vi "AuMT8852B Password.vi"(5 "New password (0)":i32, 7 "Old password (0)":i32, 8 "error in (no error)":errorcluster, 11 "VISA session":refnum<visa-resource-name>) -> (0 "error out":errorcluster, 2 "error code":i32, 3 "VISA session out":refnum<visa-resource-name>)   [LabVIEW 2017]
doc: "Anritsu MT8852B Bluetooth Tester\n\nSets the password used to lock scripts. A password is an integer from 1 to 65535.\n\nINPUTS\nOld password - the MT8850 requires the current password before it will accept a new one.\nNew password - password to be used for locking/unlocking scripts."
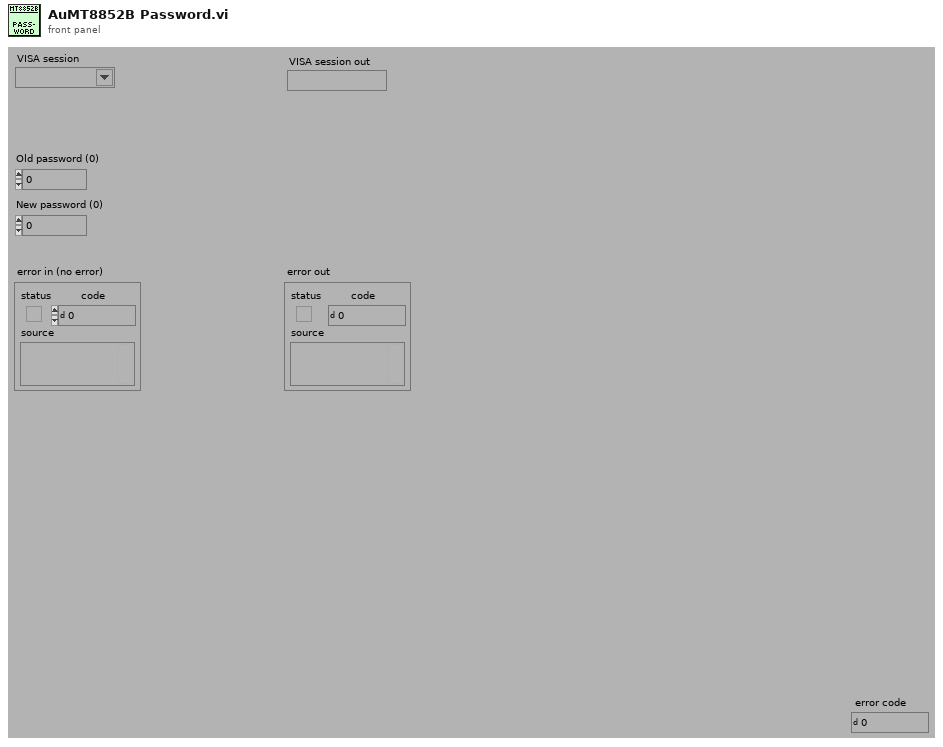
[diagram p1: front panel]
types:
  T1 = enum16{"Simulate", "Range check", "Cache", "Query instrument status"}
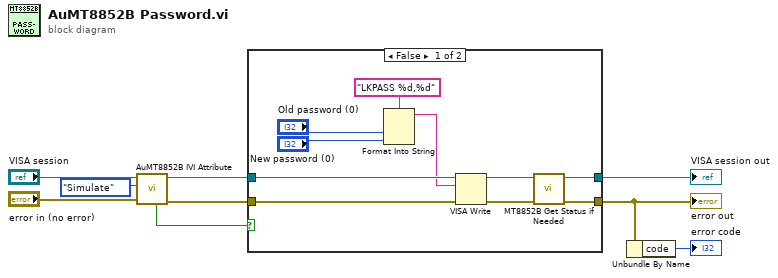
[diagram p0: block diagram]
diagram:
  n1 = call <instrlib>:"AuMT8852B IVI Attribute.vi"("error in (no error)"="error in (no error)", "Flag (Simulate)"=T1."Simulate", "VISA session"="VISA session") -> ("error out"=w4:errorcluster, "VISA session out"=w6:refnum<visa-resource-name>, "Value out"=w3:bool)  [unwired: 6 in]
  n2 = case shown="False" w3 {
    tunnel: [w19 w21] -> w1
    tunnel: [w18 w20] -> w9
    tunnel: w6 -> [w15 w20]
    tunnel: w4 -> [w14 w21]
    frame False {
      n3 = Format Into String(format string="LKPASS %d,%d" ("Format String"), "Old password (0)", "New password (0)") -> (resulting string=w10:string)  [unwired: 2 in, 1 out]
      n4 = VISA Write(VISA resource name=w15, write buffer=w10, error in (no error)=w14) -> (VISA resource name out=w17:refnum<visa-resource-name>, error out=w16:errorcluster)  [unwired: 1 out]
      n5 = call <instrlib>:"MT8852B Get Status if Needed.vi"("error in (no error)"=w16, "VISA session"=w17) -> ("error out"=w19:errorcluster, "VISA session out"=w18:refnum<visa-resource-name>)  [unwired: 8 in]
    }
    frame True {
    }
  }
  "error out" <- w1
  "VISA session out" <- w9
  n6 = Unbundle By Name(w1) -> ("code"=→"error code":i32)
